vi "HighTc_VI_2013c.vi"() -> ()   [LabVIEW 2013]
uses:
  <vilib>/Utility/file.llb/Write To Spreadsheet File (DBL).vi
panel:
  out "LockIn Y channel":cluster{i32[], dbl[]}(graph)
  out "Y Channel":dbl format="%.4e"
  out "X Channel":dbl format="%.4e"
  out "LockIn X channel":cluster{i32[], dbl[]}(graph)
  in  "Wait time (s)":dbl format="%.2f"
  in  "GPIB Lock-In":string="20"
  out "Multimeter":cluster{i32[], dbl[]}(graph)={[0, 1, 2, 3, 4], [-1.202e-05, 2.1101e-05, 6.903e-06, 1.2217e-05, -2.638e-06]}
  in  "?":bool
  in  "GPIB Multimeter":string="22"
  out "Multimeter":dbl=-2.638e-06 format="%.4e"
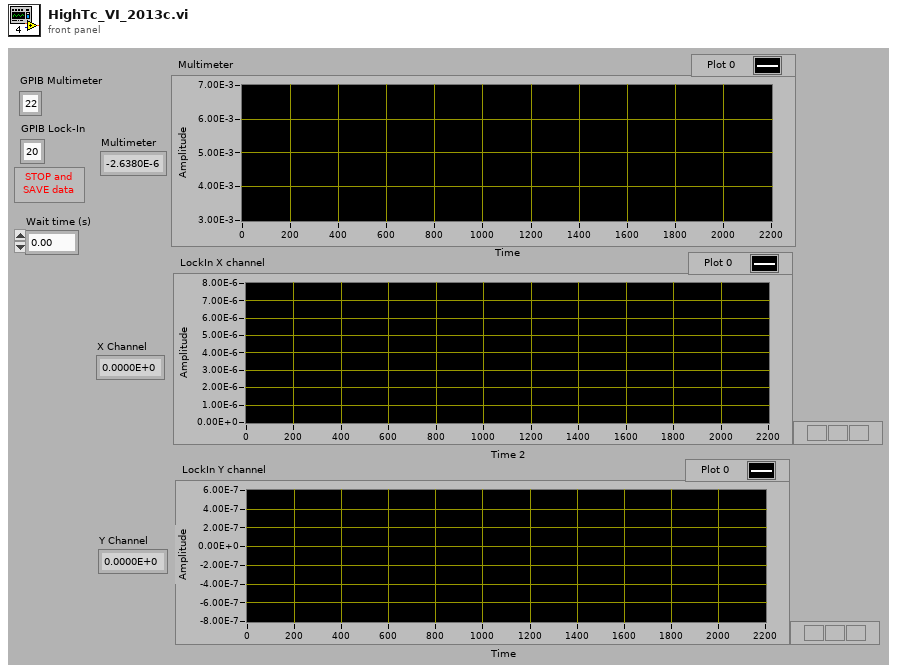
[diagram p1: front panel]
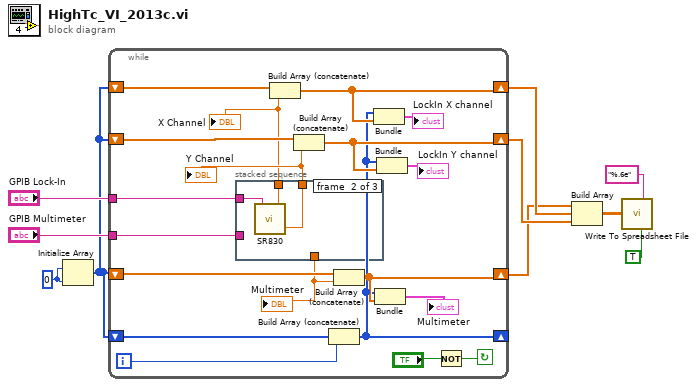
[diagram p0: block diagram]
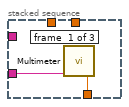
[diagram p2: hidden frame]
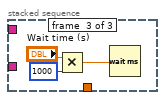
[diagram p3: hidden frame]
diagram:
  w10 = 0
  n1 = Initialize Array(w10, w10) -> (w4:i32[])
  n2 = while {
    shift-right: [w23] -> w1
    shift-left: w4 -> [w27]
    shift-right: [w12] -> _
    shift-left: w4 -> [w26]
    shift-right: [w13] -> w3
    shift-left: w4 -> [w22]
    shift-right: [w15] -> w2
    shift-left: w4 -> [w21]
    tunnel: "GPIB Multimeter" -> [w20]
    tunnel: "GPIB Lock-In" -> [w18]
    i -> [w25]
    stop <- w28 continue-if-true
    n3 = stacked-sequence {
      tunnel: w20 -> [w31 _ _]
      tunnel: [w30 _ _] -> w19
      tunnel: w18 -> [_ w34 _]
      tunnel: [_ w33 _] -> w16
      tunnel: [_ w32 _] -> w17
      frame #0 {
        n4 = call "Multimeter.vi"("GPIB address"=w31) -> ("DC Voltage"=w30:dbl)
      }
      frame #1 {
        n5 = call "SR830.vi"("GPIB address"=w34) -> ("x channel"=w33:dbl, "y channel"=w32:dbl)
      }
      frame #2 {
        n6 = Multiply(x="Wait time (s)", y=1000) -> (x*y=w35:dbl)
        n7 = Wait (ms)(milliseconds to wait=w35) -> ()  [unwired: 1 out]
      }
    }
    "Multimeter" <- w19
    "X Channel" <- w16
    "Y Channel" <- w17
    n8 = Build Array (concatenate)(w22, w16) -> (w13:dbl[])
    n9 = Build Array (concatenate)(w21, w17) -> (w15:dbl[])
    n10 = Build Array (concatenate)(w26, w25) -> (w12:i32[])
    n11 = Build Array (concatenate)(w27, w19) -> (w23:dbl[])
    n12 = Bundle(w12, w13) -> (→"LockIn X channel":cluster{i32[], dbl[]})  [unwired: 1 in]
    n13 = Bundle(w12, w23) -> (→"Multimeter":cluster{i32[], dbl[]})  [unwired: 1 in]
    n14 = Bundle(w12, w15) -> (→"LockIn Y channel":cluster{i32[], dbl[]})  [unwired: 1 in]
    n15 = Not(x="?") -> (.not. x?=w28:bool)
  }
  n16 = Build Array(w1, w3, w2) -> (w7:dbl[][])
  n17 = call-poly <vilib>:"Write To Spreadsheet File.vi"("transpose? (no:F)"=TRUE, "format (%.3f)"="%.6e", "2D data"=w7) -> ()  [unwired: 5 in, 1 out]
